vi "Read Id.vi"(8 "error in (no error)":errorcluster, 11 "WriteCommand in":refnum<class "WriteCommand.lvclass">) -> (0 "error out":errorcluster, 2 "Id":string, 3 "WriteCommand out":refnum<class "WriteCommand.lvclass">)   [LabVIEW 2023, in "HAF.lvlib" / "WriteCommand.lvclass"]
doc: "Returns the Command's unique id. If not set, a UUID is generated and stored."
uses:
  WriteCommand.lvclass
  WriteCommand.lvclass/WriteCommand.ctl
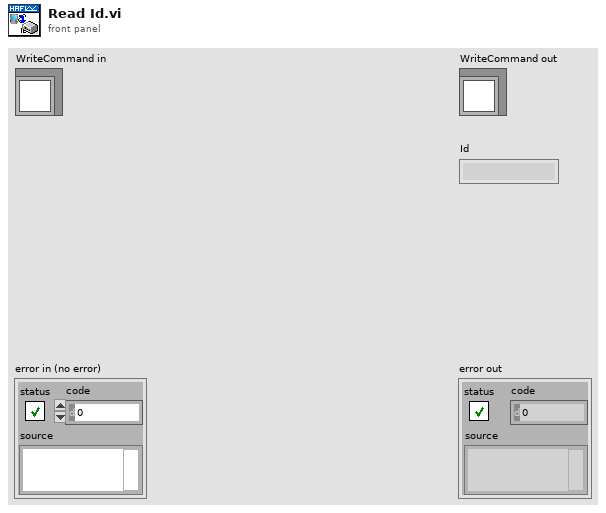
[diagram p1: front panel]
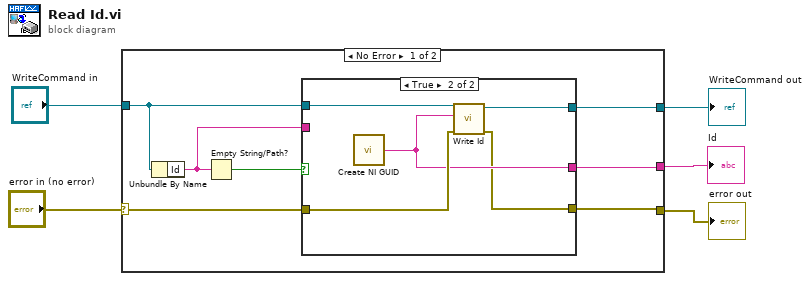
[diagram p0: block diagram]
diagram:
  n1 = case shown="No Error" "error in (no error)" {
    selector: "error in (no error)" -> [w10 w21]
    tunnel: [w6 w21] -> w4
    tunnel: [w8 w22] -> w2
    tunnel: "WriteCommand in" -> [w9 w22]
    tunnel: [w7 _] -> w1
    frame No Error {
      n2 = Unbundle By Name(w9) -> ("Id"=w11:string)
      n3 = Empty String/Path?(string/path=w11) -> (empty?=w12:bool)
      n4 = case shown="True" w12 {
        tunnel: w11 -> [w15 _]
        tunnel: w10 -> [w14 w18]
        tunnel: w9 -> [w13 w20]
        tunnel: [w13 w19] -> w8
        tunnel: [w15 w17] -> w7
        tunnel: [w14 w16] -> w6
        frame False {
        }
        frame True {
          n5 = call <vilib>:"Create NI GUID.vi"() -> ("NI GUID"=w17:string)
          n6 = call-dynamic "Write Id.vi"("error in (no error)"=w18, "Id"=w17, "WriteCommand in"=w20) -> ("error out"=w16:errorcluster, "WriteCommand out"=w19:refnum<class "WriteCommand.lvclass">)  [unwired: 7 in]
        }
      }
    }
    frame Error {
    }
  }
  "error out" <- w4
  "WriteCommand out" <- w2
  "Id" <- w1
